vi "textParse.vi"(8 "error in (no error)":errorcluster, 10 "file name":string, 11 "base path":path=path "C:/specsheetsController/Sheets/Controller") -> (0 "error out":errorcluster, 2 "all rows":string[][](array[string]), 3 "appended path":path)   [LabVIEW 2018]
uses:
  <vilib>/Utility/file.llb/Read Delimited Spreadsheet (string).vi
panel:
  out "LED Frequency Max":string
  out "LED Frequency Min":string
  out "LED Frequency (Charge)":string
  out "LED Frequency (Limit)":string
  out "LED Frequency (Foldback)":string
  out "HV Bus Voltage(@10% PWM)":string
  out "HV Bus Tol. Min":string
  out "HV Bus Tol. Max":string
  out "Speed Pot Voltage Low(@85% PWM)":string
  out "Speed Pot Voltage Mid(@85% PWM)":string
  out "Speed Pot Voltage High(@85% PWM)":string
  out "Speed Pot Voltage Tol. Min":string
  out "Speed Pot Voltage Tol. Max":string
  out "Ircomp(@70% PWM)":string
  out "Current Running Tol. Min":string
  out "Current Running Tol. Max":string
  out "Current Limit(@45% PWM)":string
  out "Sense Voltage Tol. Max":string
  out "Sense Voltage Tol. Min":string
  out "Sense Voltage":string
  out "Allowable Power Interuption":string
  out "Voltage FET Driver Tol. Max":string
  out "Voltage FET Driver Tol. Min":string
  out "Voltage FET Driver":string
  out "Voltage Micro Tol. Max":string
  out "Voltage Micro Tol. Min":string
  out "Voltage Micro":string
  out "Rated Output Current Tol. Max":string
  out "Rated Output Current Tol. Min":string
  out "Rated Output Current":string
  out "Ripple/Noise Tol. Max":string
  out "Ripple/Noise Tol. Min":string
  out "Ripple/Noise":string
  out "Voltage Output Tol. Max":string
  out "Voltage  Output Tol. Min":string
  out "Voltage Output":string
  out "Max Input Current":string
  out "Input Current":string
  out "Input Voltage Tol. Max":string
  out "Input Voltage Tol. Min":string
  out "Input Voltage":string
  out "Firmware":string
  out "Part Number":string
  out "Part Name":string
  # "Global variables"
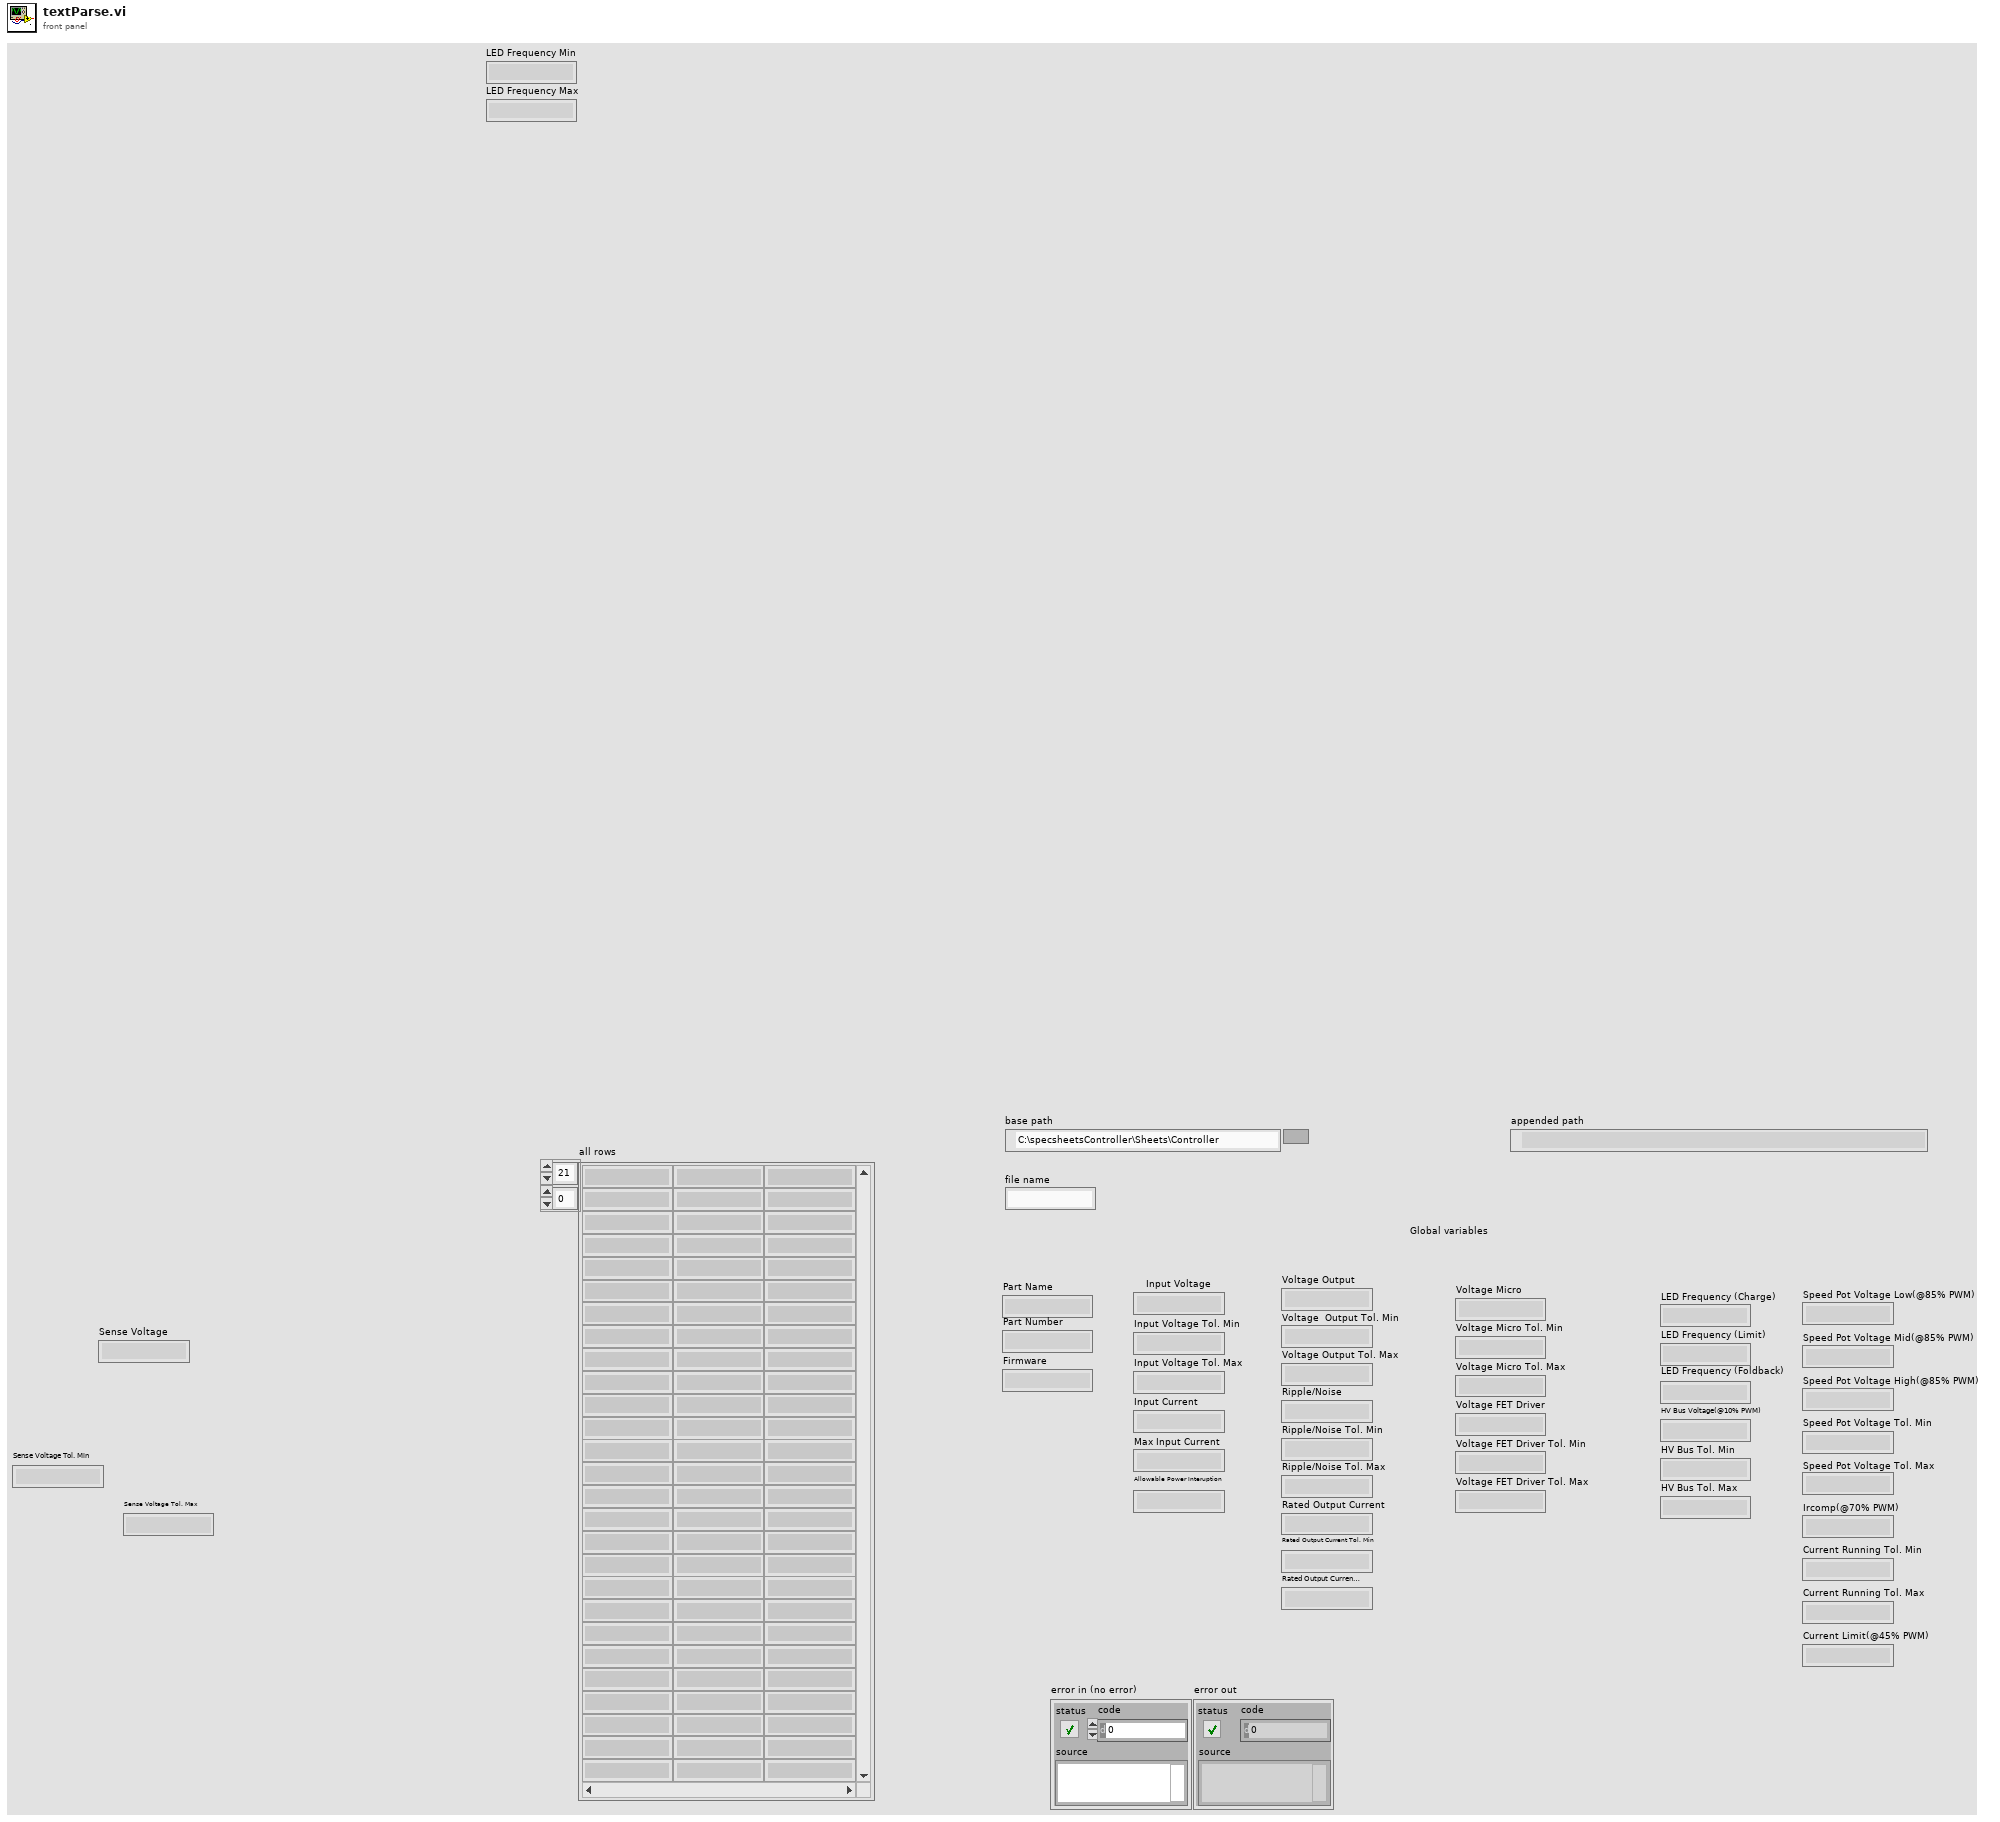
[diagram p1: front panel]
types:
  T1 = enum16{"Main", "In Primary", "Secondary", "Out Primary", "Motor Drive", ""}
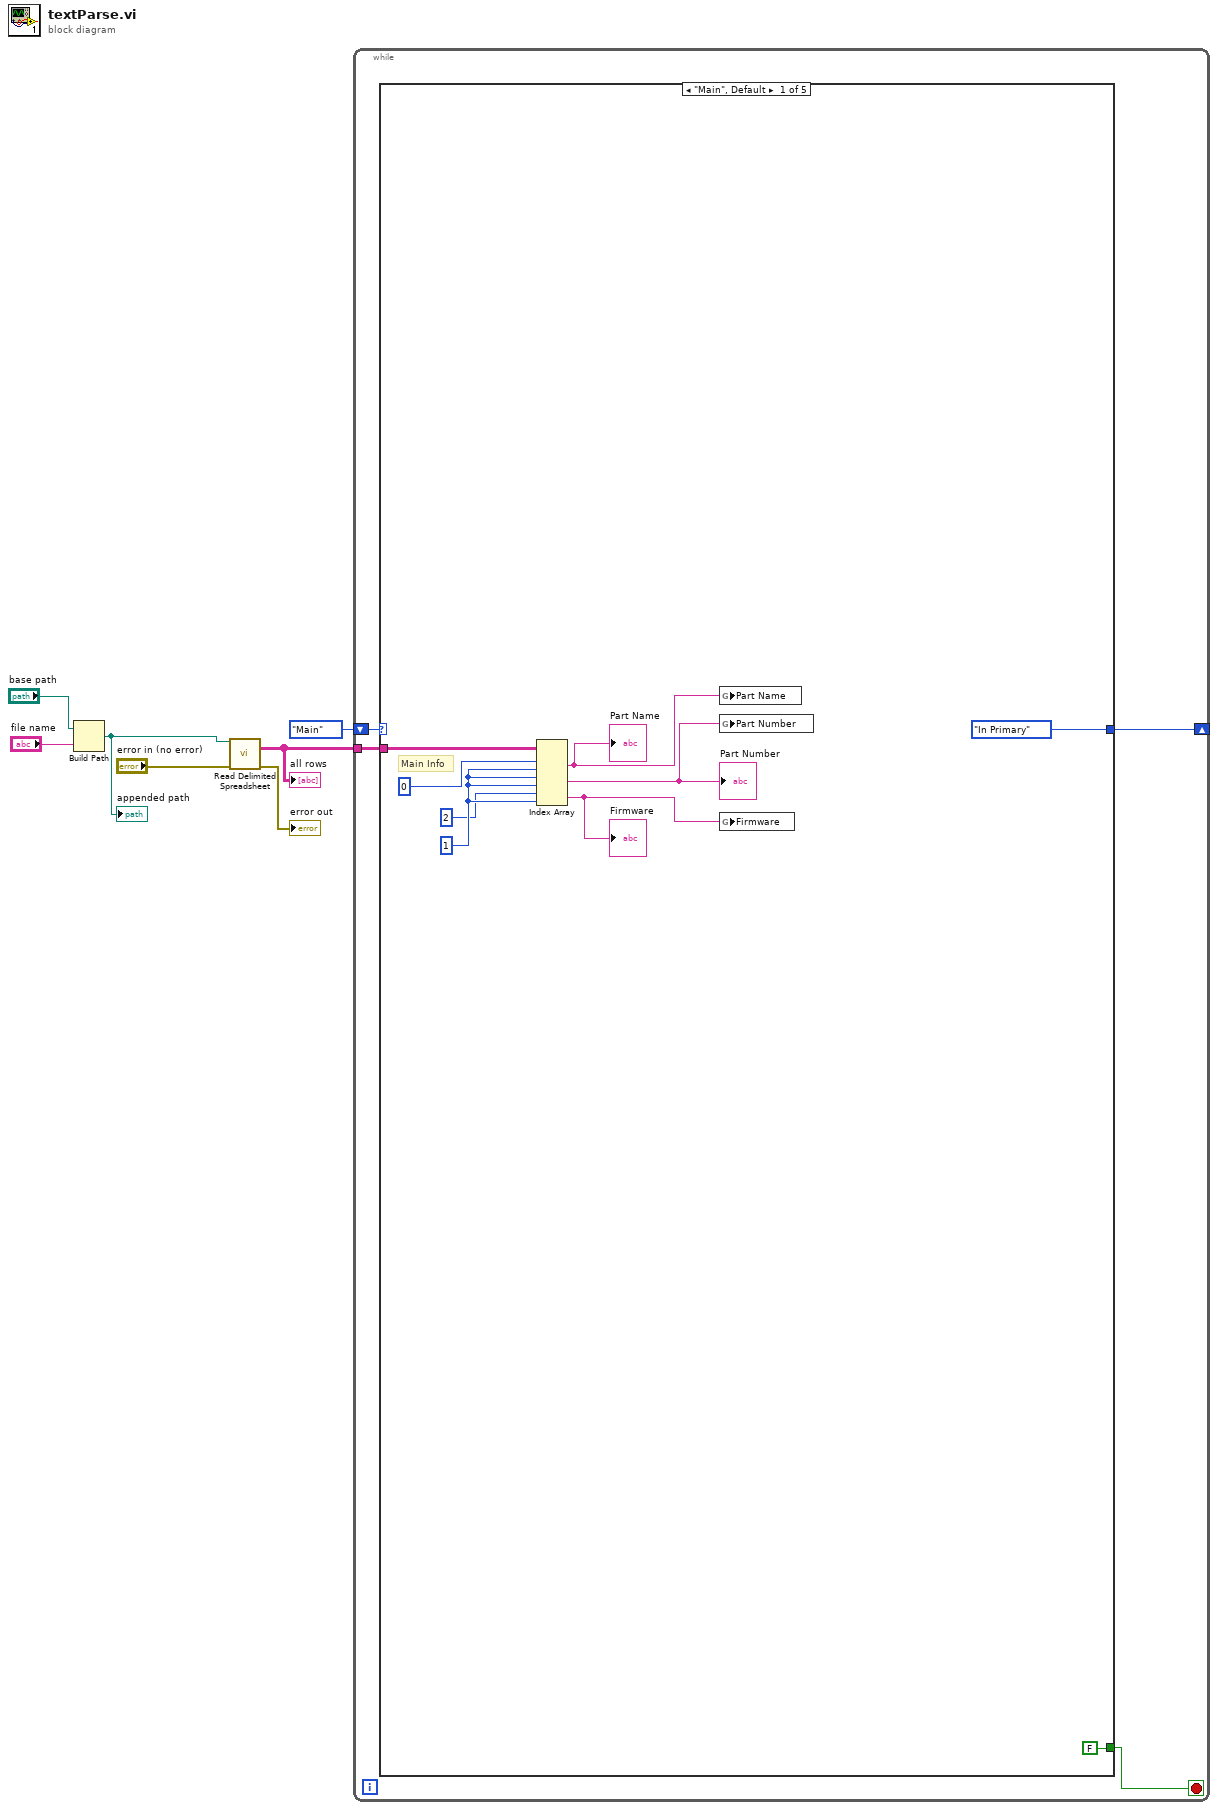
[diagram p0: block diagram]
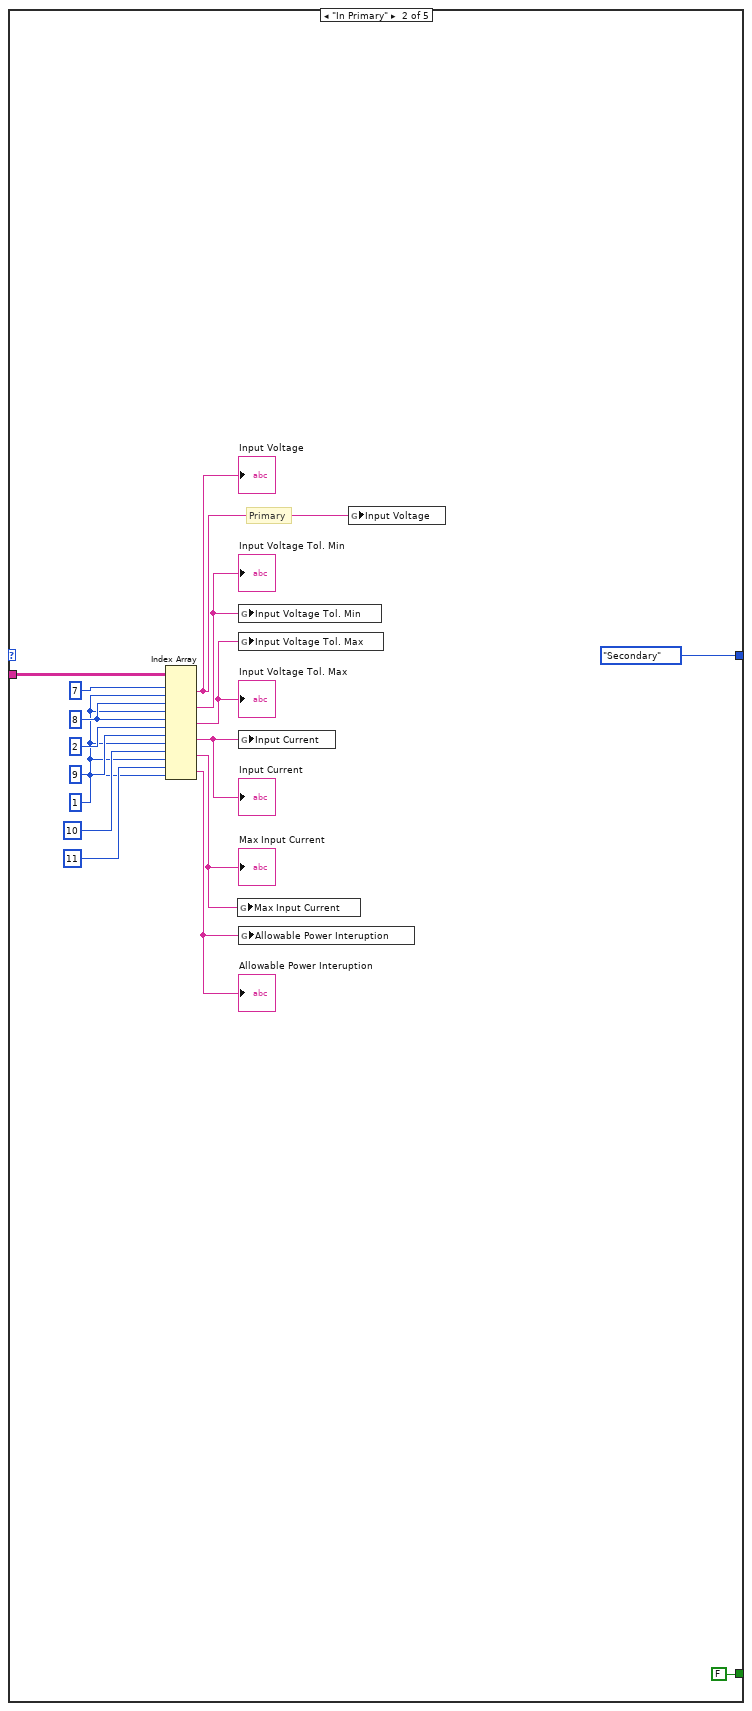
[diagram p2: hidden frame]
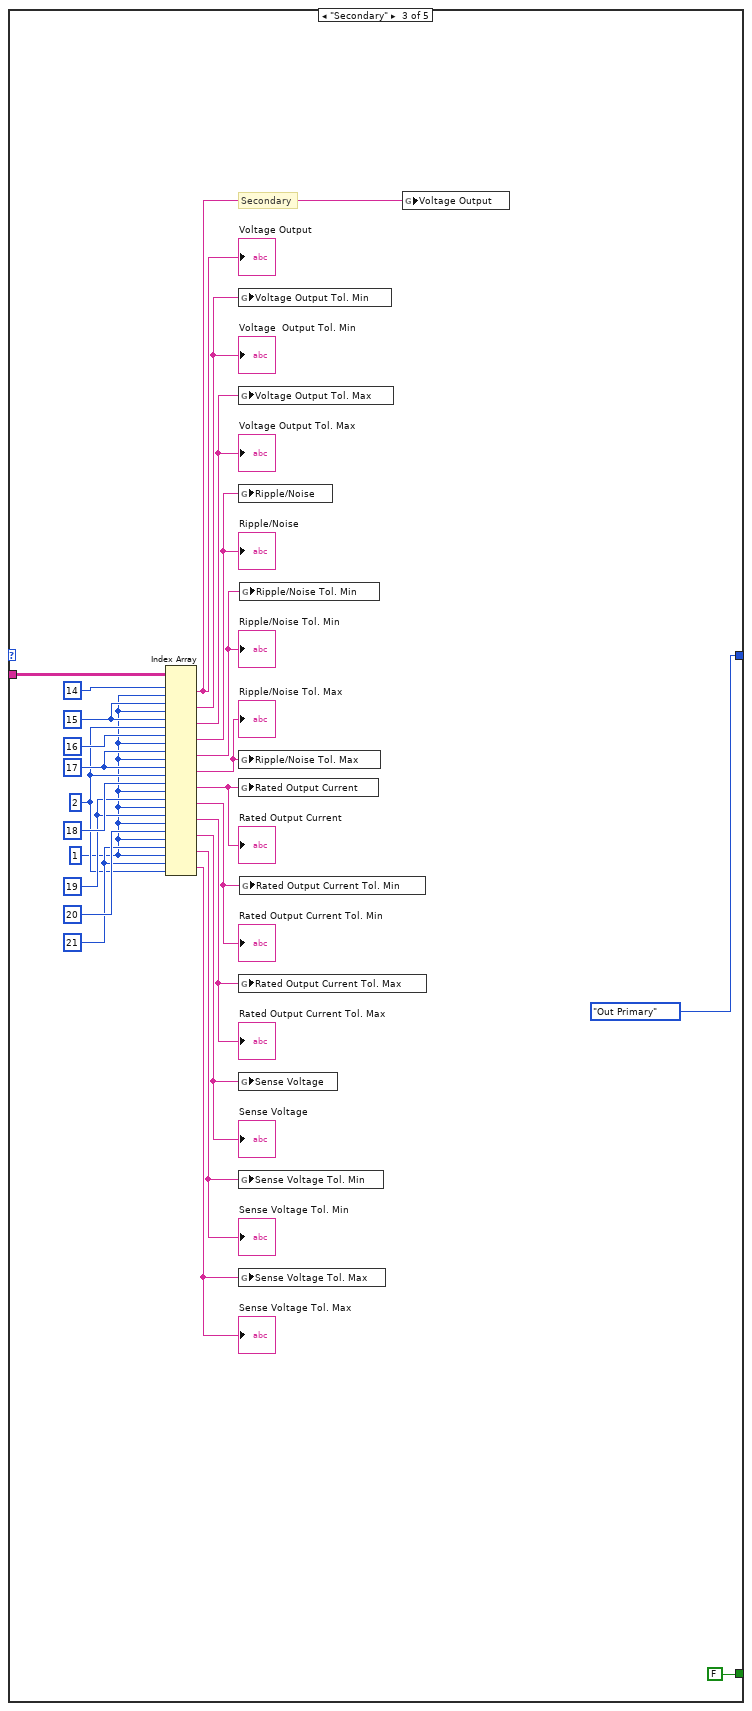
[diagram p3: hidden frame]
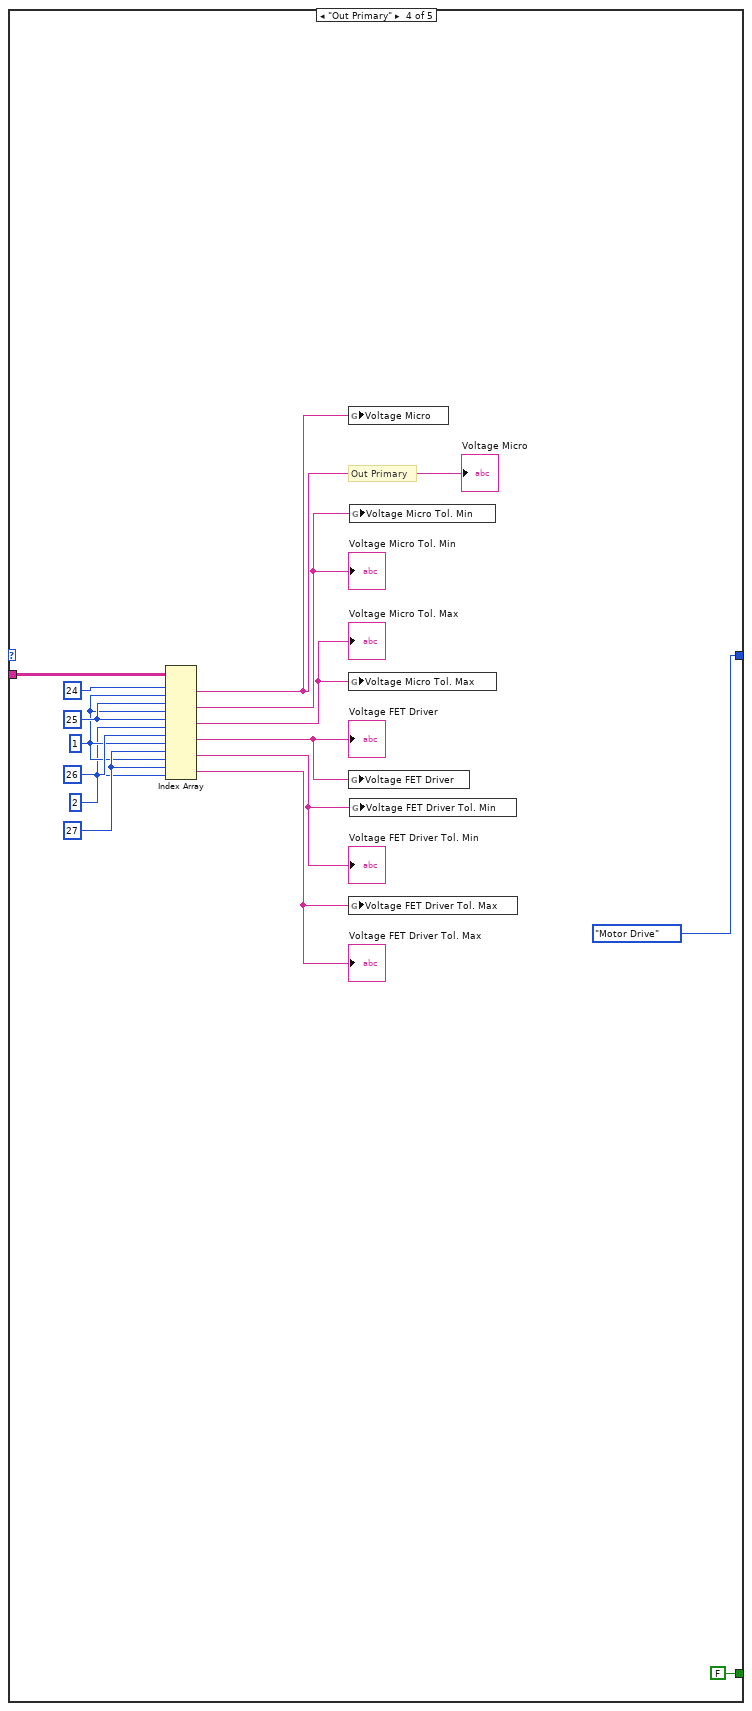
[diagram p4: hidden frame]
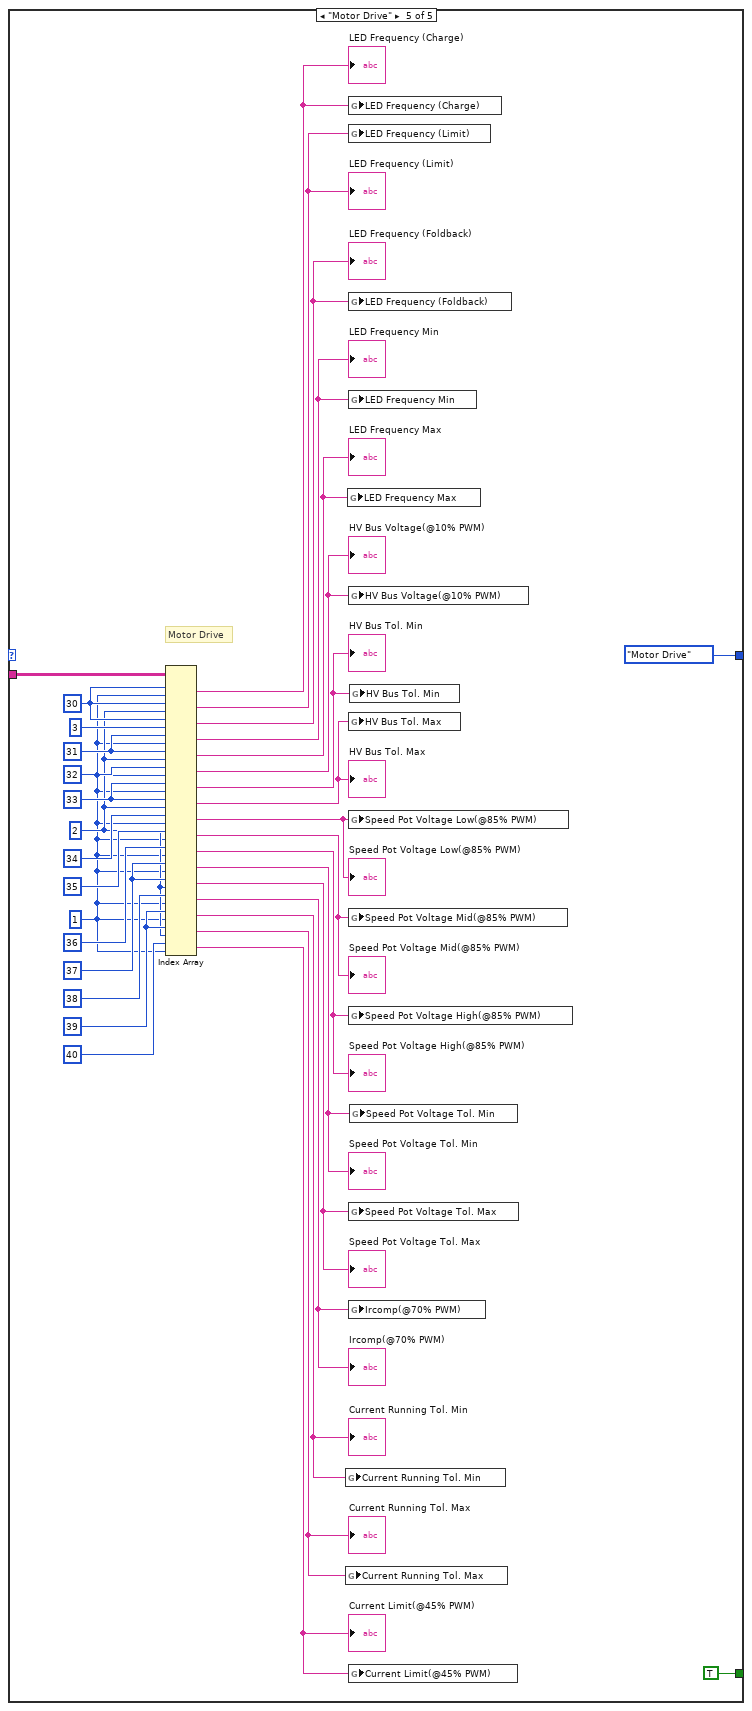
[diagram p5: hidden frame]
diagram:
  n1 = Build Path(base path="base path", name or relative path="file name") -> (appended path=w5:path)
  "appended path" <- w5
  n2 = call-poly <vilib>:"Read Delimited Spreadsheet.vi"("file path (dialog if empty)"=w5, "error in (no error)"="error in (no error)") -> ("all rows"=w2:string[][], "error out"=→"error out":errorcluster)  [unwired: 8 in, 4 out]
  "all rows" <- w2
  n3 = while {
    shift-right: [w11] -> _
    shift-left: T1."Main" -> [w9]
    tunnel: w2 -> [w10]
    stop <- w8 stop-if-true
    n4 = case shown="\"Main\", Default" w9 {
      tunnel: w10 -> [w14 w25 w46 w66 w110]
      tunnel: [T1."In Primary" T1."Secondary" T1."Out Primary" T1."Motor Drive" T1."Motor Drive"] -> w11
      tunnel: [FALSE FALSE FALSE FALSE TRUE] -> w8
      frame "Main", Default {
        w16 = 1
        # "Main Info"
        n5 = Index Array(array=w14, index (row) #1=0 ("index (row)"), index (col) #1=w16, index (row) #2=w16, index (col) #2=w16, index (row) #3=2 ("index (row)"), index (col) #3=w16) -> (element #1=w18:string, element #2=w20:string, element #3=w19:string)
        "Part Name" <- w18
        "Part Number" <- w20
        "Firmware" <- w19
        n6 = global write "Global textParse.vi" "Part Name"(w18) -> ()
        n7 = global write "Global textParse.vi" "Part Number"(w20) -> ()
        n8 = global write "Global textParse.vi" "Firmware"(w19) -> ()
      }
      frame "In Primary" {
        w29 = 8
        w23 = 1
        # "Primary"
        n9 = Index Array(array=w25, index (row) #1=7, index (col) #1=w23, index (row) #2=w29, index (col) #2=w23, index (row) #3=w29, index (col) #3=2, index (row) #4=9, index (col) #4=w23, index (row) #5=10, index (col) #5=w23, index (row) #6=11, index (col) #6=w23) -> (element #1=w31:string, element #2=w32:string, element #3=w33:string, element #4=w34:string, element #5=w35:string, element #6=w36:string)
        "Input Voltage" <- w31
        "Input Voltage Tol. Min" <- w32
        "Input Voltage Tol. Max" <- w33
        "Input Current" <- w34
        "Max Input Current" <- w35
        "Allowable Power Interuption" <- w36
        n10 = global write "Global textParse.vi" "Max Input Current"(w35) -> ()
        n11 = global write "Global textParse.vi" "Input Voltage Tol. Min"(w32) -> ()
        n12 = global write "Global textParse.vi" "Input Voltage Tol. Max"(w33) -> ()
        n13 = global write "Global textParse.vi" "Input Current"(w34) -> ()
        n14 = global write "Global textParse.vi" "Allowable Power Interuption"(w36) -> ()
        n15 = global write "Global textParse.vi" "Input Voltage"(w31) -> ()
      }
      frame "Secondary" {
        w44 = 21 ("index (row)")
        w47 = 19 ("index (row)")
        w42 = 1
        w43 = 2
        w49 = 17 ("index (row) 15")
        w51 = 15 ("index (row) 13")
        # "Secondary"
        n16 = Index Array(array=w46, index (row) #1=14 ("index (row) 12"), index (col) #1=w42, index (row) #2=w51, index (col) #2=w42, index (row) #3=w51, index (col) #3=w43, index (row) #4=16 ("index (row) 14"), index (col) #4=w42, index (row) #5=w49, index (col) #5=w42, index (row) #6=w49, index (col) #6=w43, index (row) #7=18 ("index (row) 19"), index (col) #7=w42, index (row) #8=w47, index (col) #8=w42, index (row) #9=w47, index (col) #9=w42, index (row) #10=20 ("index (row)"), index (col) #10=w42, index (row) #11=w44, index (col) #11=w42, index (row) #12=w44, index (col) #12=w43) -> (element #1=w53:string, element #2=w54:string, element #3=w55:string, element #4=w56:string, element #5=w57:string, element #6=w58:string, element #7=w59:string, element #8=w60:string, element #9=w61:string, element #10=w41:string, element #11=w40:string, element #12=w39:string)
        "Voltage Output" <- w53
        "Voltage  Output Tol. Min" <- w54
        "Voltage Output Tol. Max" <- w55
        "Ripple/Noise" <- w56
        "Ripple/Noise Tol. Min" <- w57
        "Ripple/Noise Tol. Max" <- w58
        "Rated Output Current" <- w59
        "Rated Output Current Tol. Min" <- w60
        "Rated Output Current Tol. Max" <- w61
        "Sense Voltage" <- w41
        "Sense Voltage Tol. Min" <- w40
        "Sense Voltage Tol. Max" <- w39
        n17 = global write "Global textParse.vi" "Voltage Output Tol. Min"(w54) -> ()
        n18 = global write "Global textParse.vi" "Voltage Output Tol. Max"(w55) -> ()
        n19 = global write "Global textParse.vi" "Ripple/Noise"(w56) -> ()
        n20 = global write "Global textParse.vi" "Ripple/Noise Tol. Max"(w58) -> ()
        n21 = global write "Global textParse.vi" "Rated Output Current"(w59) -> ()
        n22 = global write "Global textParse.vi" "Rated Output Current Tol. Max"(w61) -> ()
        n23 = global write "Global textParse.vi" "Sense Voltage"(w41) -> ()
        n24 = global write "Global textParse.vi" "Sense Voltage Tol. Min"(w40) -> ()
        n25 = global write "Global textParse.vi" "Sense Voltage Tol. Max"(w39) -> ()
        n26 = global write "Global textParse.vi" "Ripple/Noise Tol. Min"(w57) -> ()
        n27 = global write "Global textParse.vi" "Rated Output Current Tol. Min"(w60) -> ()
        n28 = global write "Global textParse.vi" "Voltage Output"(w53) -> ()
      }
      frame "Out Primary" {
        w63 = 2
        w64 = 1
        w67 = 27 ("index (row) 27")
        w69 = 25 ("index (row) 25")
        # "Out Primary"
        n29 = Index Array "Index Array"(array=w66, index (row) #1=24 ("index (row) 24"), index (col) #1=w64, index (row) #2=w69, index (col) #2=w64, index (row) #3=w69, index (col) #3=w63, index (row) #4=26 ("index (row) 26"), index (col) #4=w64, index (row) #5=w67, index (col) #5=w64, index (row) #6=w67, index (col) #6=w63) -> (element #1=w71:string, element #2=w72:string, element #3=w73:string, element #4=w74:string, element #5=w75:string, element #6=w76:string)
        "Voltage Micro" <- w71
        "Voltage Micro Tol. Min" <- w72
        "Voltage Micro Tol. Max" <- w73
        "Voltage FET Driver" <- w74
        "Voltage FET Driver Tol. Min" <- w75
        "Voltage FET Driver Tol. Max" <- w76
        n30 = global write "Global textParse.vi" "Voltage Micro"(w71) -> ()
        n31 = global write "Global textParse.vi" "Voltage Micro Tol. Max"(w73) -> ()
        n32 = global write "Global textParse.vi" "Voltage FET Driver"(w74) -> ()
        n33 = global write "Global textParse.vi" "Voltage FET Driver Tol. Max"(w76) -> ()
        n34 = global write "Global textParse.vi" "Voltage Micro Tol. Min"(w72) -> ()
        n35 = global write "Global textParse.vi" "Voltage FET Driver Tol. Min"(w75) -> ()
      }
      frame "Motor Drive" {
        w97 = 2
        w96 = 1
        w99 = 39
        w101 = 37
        w105 = 33 ("index (row) 28")
        w107 = 31 ("index (row) 25")
        w108 = 30 ("index (row) 24")
        # "Motor Drive"
        n36 = Index Array "Index Array"(array=w110, index (row) #1=w108, index (col) #1=w96, index (row) #2=w108, index (col) #2=w97, index (row) #3=w108, index (col) #3=3, index (row) #4=w107, index (col) #4=w96, index (row) #5=w107, index (col) #5=w97, index (row) #6=32 ("index (row) 26"), index (col) #6=w96, index (row) #7=w105, index (col) #7=w96, index (row) #8=w105, index (col) #8=w97, index (row) #9=34 ("index (row) 29"), index (col) #9=w96, index (row) #10=35, index (col) #10=w96, index (row) #11=36 ("index (row) 30"), index (col) #11=w96, index (row) #12=w101, index (col) #12=w96, index (row) #13=w101, index (col) #13=w97, index (row) #14=38, index (col) #14=w96, index (row) #15=w99, index (col) #15=w96, index (row) #16=w99, index (col) #16=w97, index (row) #17=40, index (col) #17=w96) -> (element #1=w95:string, element #2=w94:string, element #3=w93:string, element #4=w92:string, element #5=w91:string, element #6=w90:string, element #7=w89:string, element #8=w88:string, element #9=w87:string, element #10=w86:string, element #11=w85:string, element #12=w84:string, element #13=w83:string, element #14=w82:string, element #15=w81:string, element #16=w80:string, element #17=w79:string)
        "LED Frequency (Charge)" <- w95
        "LED Frequency (Limit)" <- w94
        "LED Frequency (Foldback)" <- w93
        "HV Bus Voltage(@10% PWM)" <- w90
        "HV Bus Tol. Min" <- w89
        "HV Bus Tol. Max" <- w88
        "Speed Pot Voltage Low(@85% PWM)" <- w87
        "Speed Pot Voltage Mid(@85% PWM)" <- w86
        "Speed Pot Voltage High(@85% PWM)" <- w85
        "Speed Pot Voltage Tol. Min" <- w84
        "Speed Pot Voltage Tol. Max" <- w83
        "Ircomp(@70% PWM)" <- w82
        "Current Running Tol. Min" <- w81
        "Current Running Tol. Max" <- w80
        "Current Limit(@45% PWM)" <- w79
        "LED Frequency Min" <- w92
        "LED Frequency Max" <- w91
        n37 = global write "Global textParse.vi" "Current Running Tol. Min"(w81) -> ()
        n38 = global write "Global textParse.vi" "Current Running Tol. Max"(w80) -> ()
        n39 = global write "Global textParse.vi" "LED Frequency Max"(w91) -> ()
        n40 = global write "Global textParse.vi" "LED Frequency (Charge)"(w95) -> ()
        n41 = global write "Global textParse.vi" "LED Frequency (Limit)"(w94) -> ()
        n42 = global write "Global textParse.vi" "LED Frequency (Foldback)"(w93) -> ()
        n43 = global write "Global textParse.vi" "LED Frequency Min"(w92) -> ()
        n44 = global write "Global textParse.vi" "HV Bus Voltage(@10% PWM)"(w90) -> ()
        n45 = global write "Global textParse.vi" "HV Bus Tol. Max"(w88) -> ()
        n46 = global write "Global textParse.vi" "Speed Pot Voltage Low(@85% PWM)"(w87) -> ()
        n47 = global write "Global textParse.vi" "Speed Pot Voltage Mid(@85% PWM)"(w86) -> ()
        n48 = global write "Global textParse.vi" "Speed Pot Voltage High(@85% PWM)"(w85) -> ()
        n49 = global write "Global textParse.vi" "Speed Pot Voltage Tol. Max"(w83) -> ()
        n50 = global write "Global textParse.vi" "Ircomp(@70% PWM)"(w82) -> ()
        n51 = global write "Global textParse.vi" "Current Limit(@45% PWM)"(w79) -> ()
        n52 = global write "Global textParse.vi" "HV Bus Tol. Min"(w89) -> ()
        n53 = global write "Global textParse.vi" "Speed Pot Voltage Tol. Min"(w84) -> ()
      }
    }
  }
